vi "#183_MAV_MSG_AUTOPILOT_VERSION_REQUEST_ENCODE.vi"(10 "packet_sequence_in":u8, 11 "AUTOPILOT_VERSION_REQUEST":T1={"self"={"system_id"=255, "component_id"=190}, "target_system"=1, "target_component"=1}) -> (2 "packet_sequence_out":u8, 3 "mavlink_buffer_out":u8[](array[numeric]))   [LabVIEW 2023]
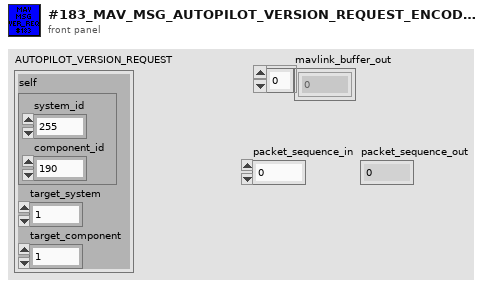
[diagram p1: front panel]
types:
  T1 = cluster{"self":cluster{"system_id":u8, "component_id":u8}, "target_system":u8, "target_component":u8}
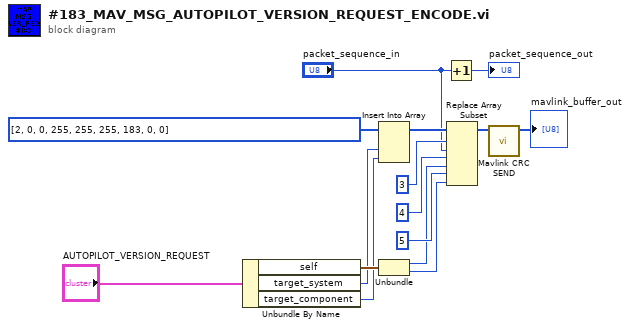
[diagram p0: block diagram]
diagram:
  n1 = Unbundle By Name("AUTOPILOT_VERSION_REQUEST") -> ("self"=w8:cluster{"system_id":u8, "component_id":u8}, "target_system"=w3:u8, "target_component"=w2:u8)
  n2 = Insert Into Array(array=u8[] [2, 0, 0, 255, 255, 255, 183, 0, 0], new element #1=w3, new element #2=w2) -> (w14:u8[])  [unwired: 1 in]
  n3 = Unbundle(w8) -> ("system_id"=w7:u8, "component_id"=w6:u8)
  n4 = Increment(x="packet_sequence_in") -> (x+1=→"packet_sequence_out":u8)
  n5 = Replace Array Subset(array=w14, new element #1="packet_sequence_in", index #1=3 ("index"), new element #2=w7, index #2=4 ("index"), new element #3=w6, index #3=5 ("index")) -> (w4:u8[])
  n6 = call "Mavlink CRC SEND.vi"("Byte In"=w4) -> ("Output Byte"=→"mavlink_buffer_out":u8[])  [unwired: 10 in]
